vi "Remote Panel Methods Client.vi"() -> ()   [LabVIEW 2023]
doc: "This VI illustrates how to programmatically connect to a remote front panel. A connection is established to the specified VI and control can also be requested. Once control is requested, the VI can only be run once since the server will close the connection automatically after one run."
panel:
  in  "Request Control":bool
  in  "Remote Panel Server Port":i32=8000
  in  "Remote Panel Server Address":string
  # "Overview: Demonstrates the use of Remote Panel methods to gain control of a target VI running on a server.\nRequirements: LabVIEW Full Development System\nInstructions:\n1. Open Remote Panel Methods Server.vi and follow the instructions on its front panel. Note that the Server VI must be running in a different instance of LabVIEW than this VI, but both LabVIEW instances must be the same version. The other instance of LabVIEW will usually be running on a different computer.\n2. Specify the Remote Panel Server Address indicated on the front panel of Remote Panel Methods Server.vi.\n3. Specify the Remote Panel Server Port indicated on the front panel of Remote Panel Methods Server.vi.\n4. Run this VI.\n5. Click the Request Control button to gain control of the target VI running on the server. In this example, the target VI is a Waveform Chart example.\n6. Run the target VI.\n7. Click Stop to stop the target VI. Note that the \"Server Regained Control\" message is displayed."
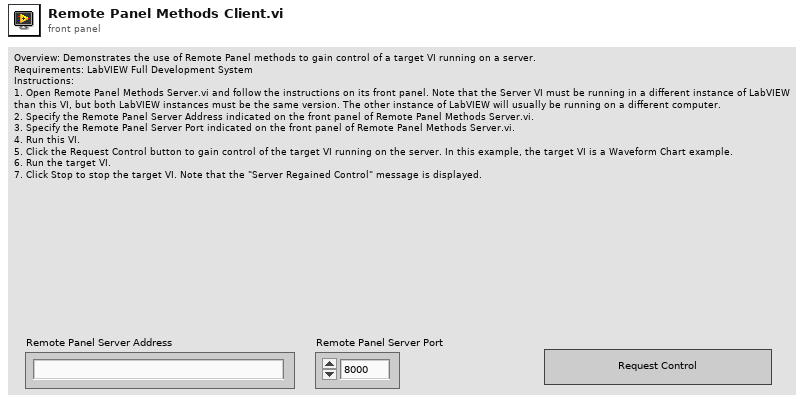
[diagram p1: front panel]
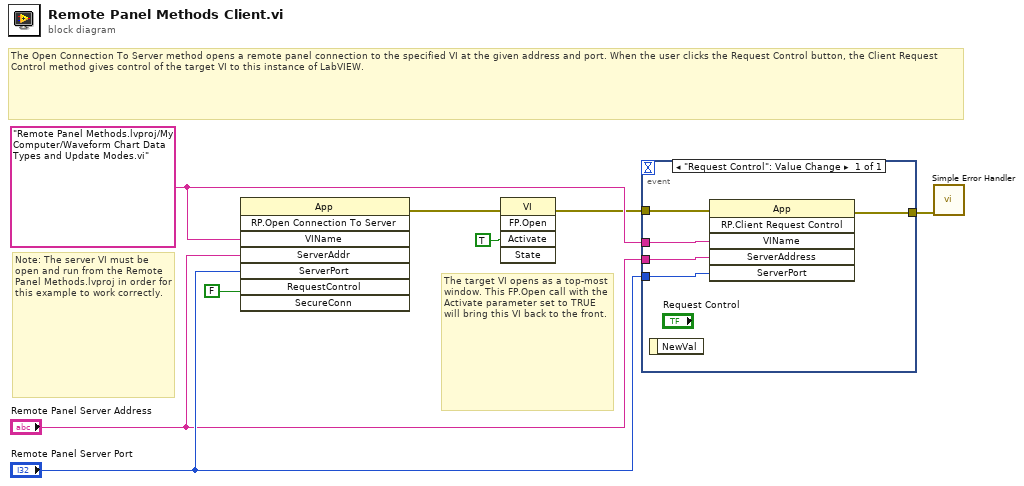
[diagram p0: block diagram]
diagram:
  w3 = "Remote Panel Methods.lvproj/My Computer/Waveform Chart Data Types and Update Modes.vi" ("VI Name")
  # "Note: The server VI must be open and run from the Remote Panel Methods.lvproj in order for this example to work correctly."
  # "The target VI opens as a top-most window. This FP.Open call with the Activate parameter set to TRUE will bring this VI back to the front."
  # "The Open Connection To Server method opens a remote panel connection to the specified VI at the given address and port. When the user clicks the Request Control button, the Client Request Control method gives control of the target VI to this instance of LabVIEW."
  n1 = invoke class="App" method="RP.Open Connection To Server"("VIName"=w3, "ServerAddr"="Remote Panel Server Address", "ServerPort"="Remote Panel Server Port", "RequestControl"=FALSE) -> (error out=w7:errorcluster)  [unwired: 4 in, 7 out]
  n2 = invoke class="VI" method="FP.Open"(error in=w7, "Activate"=TRUE ("Activate?")) -> (error out=w2:errorcluster)  [unwired: 3 in, 4 out]
  n3 = event shown="[0] \"Request Control\": Value Change" {
    selector: _ -> [_]
    dyn-events: _ -> [_]
    timeout: _ -> [_]
    tunnel: w2 -> [w13]
    tunnel: [w12] -> w6
    tunnel: "Remote Panel Server Port" -> [w11]
    tunnel: "Remote Panel Server Address" -> [w10]
    tunnel: w3 -> [w9]
    event "Request Control": Value Change {
      n4 = event-data() -> ()  [unwired: 1 in, 1 out]
      n5 = invoke class="App" method="RP.Client Request Control"(error in=w13, "VIName"=w9, "ServerAddress"=w10, "ServerPort"=w11) -> (error out=w12:errorcluster)  [unwired: 2 in, 5 out]
    }
  }
  n6 = call <vilib>:"Simple Error Handler.vi"("error in (no error)"=w6) -> ()  [unwired: 4 in, 5 out]
